vi "Get LSD.vi"(8 "error in (no error)":errorcluster caption="错误输入（无错误）", 11 "Gif Image输入":refnum<class "Gif Image.lvclass">) -> (0 "error out":errorcluster caption="错误输出", 2 "Logical Screen Descriptor":T1 {"Pack Field" format="%.0x"}, 3 "Gif Image输出":refnum<class "Gif Image.lvclass">)   [LabVIEW 2012, in "Picture Box Tools.lvlib" / "Gif Image.lvclass"]
uses:
  Gif Image.lvclass
  Control/Logical Screen Descriptor.ctl
  Gif Image.lvclass/Gif Image.ctl
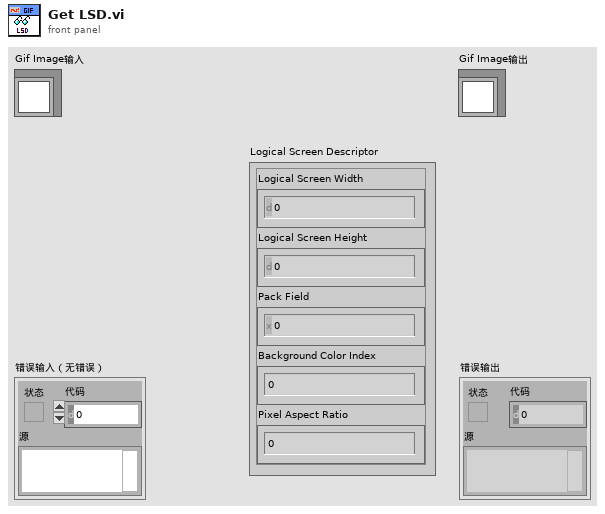
[diagram p1: front panel]
types:
  T1 = typedef "Picture Box Tools.lvlib/Gif Image.lvclass/Logical Screen Descriptor.ctl" = cluster{"Logical Screen Width":u16, "Logical Screen Height":u16, "Pack Field":u8, "Background Color Index":u8, "Pixel Aspect Ratio":u8}
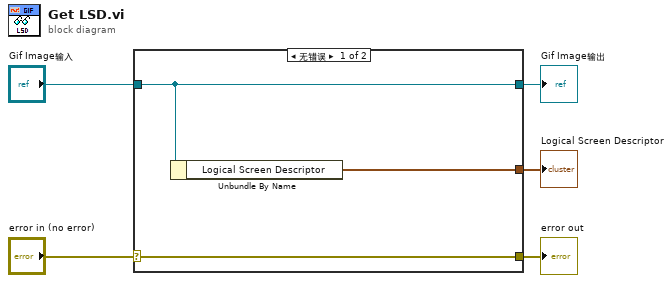
[diagram p0: block diagram]
diagram:
  n1 = case shown="无错误" "error in (no error)" {
    selector: "error in (no error)" -> [w8 w9]
    tunnel: [w8 w9] -> w4
    tunnel: [w7 w10] -> w2
    tunnel: "Gif Image输入" -> [w7 w10]
    tunnel: [w6 _] -> w1
    frame No Error {
      n2 = Unbundle By Name(w7) -> ("Logical Screen Descriptor"=w6:T1)
    }
    frame Error {
    }
  }
  "error out" <- w4
  "Gif Image输出" <- w2
  "Logical Screen Descriptor" <- w1
